vi "MAIN.vi"() -> ()   [LabVIEW 2017]
doc: "该模板用于创建生产者／消费者模式的应用程序，以事件驱动的方式，生成队列中的项。如需通过响应事件实现代码的异步执行，同时不影响用户界面的响应速度，可考虑用该模式替代“用户界面事件处理器”模式。"
uses:
  SubVIs/ctl/Status.ctl
  SubVIs/DataBaseModule/Sqlite/CBB/UpdateAllData.vi
  SubVIs/DataBaseModule/Sqlite/SQLite.lvlib
panel:
  out "stripped path":path
  out "设备Status":T1[](array[typedef])
  in  "设备明细簇":T2[](array[typedef])
  out "元素":string
  in  "选项卡控件":enum32{"主界面", "设置"}(tab)
  out "系统信息":string
  out "Status":T1
  in  "设备名称":T3
  in  "stop":bool caption="停止"
  in  "应用名称":string="InoTouchPad"
  in  "设备明细表格":string[][](table)
  in  "单台设备明细":T2
  out "数据输出":string
  in  "Enqueue Element":bool caption="元素入队列"
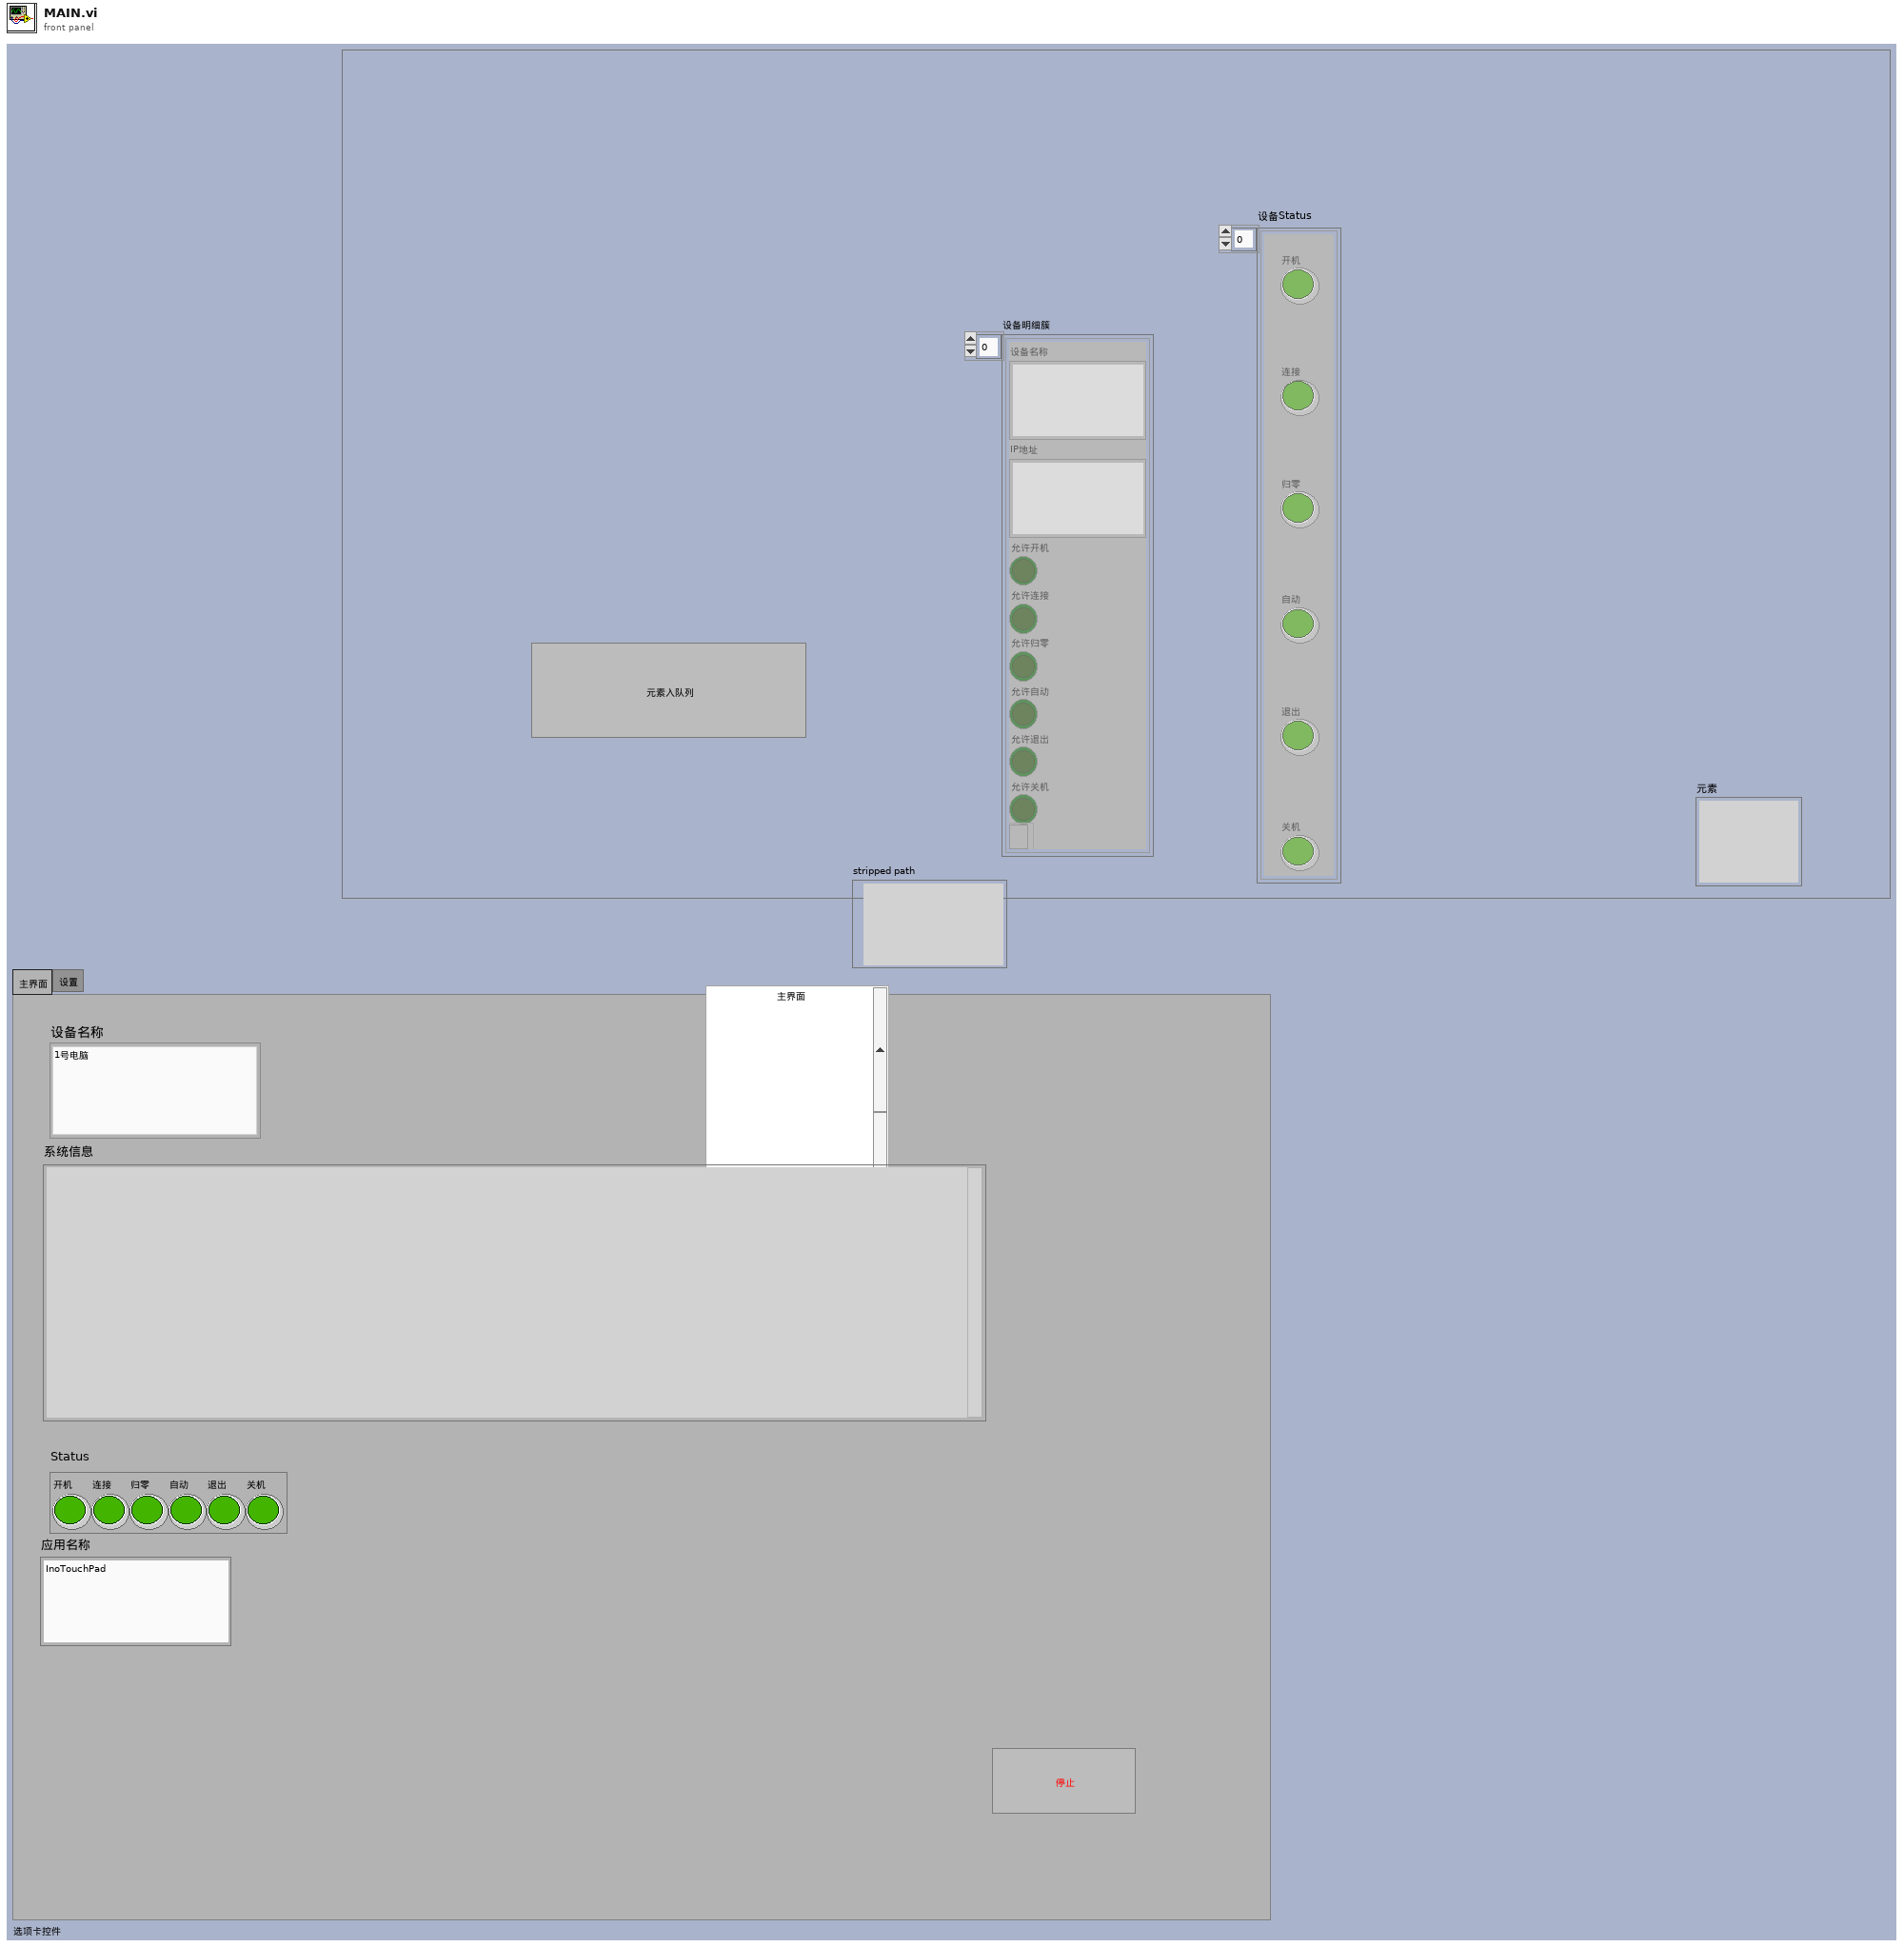
[diagram p1: front panel]
types:
  T1 = typedef "Status.ctl" = cluster{"开机":bool, "连接":bool, "归零":bool, "自动":bool, "退出":bool, "关机":bool}
  T2 = typedef "单台设备明细.ctl" = cluster{"设备名称":string, "IP地址":string, "允许开机":bool, "允许连接":bool, "允许归零":bool, "允许自动":bool, "允许退出":bool, "允许关机":bool, "connection ID":refnum<k5>}
  T3 = typedef "设备名称.ctl" = enum16{"1号电脑", "2号电脑"}
  T4 = enum32{"invalid app kind", "Development System", "Run Time System", "Student Edition", "Embedded LabVIEW", "Evaluation", "Custom"}
  T5 = typedef "界面控件引用.ctl" = cluster{"设备名称":refnum<vi>, "Status":refnum<vi>, "设备明细表格":refnum<vi>, "系统信息":refnum<vi>, "设备明细簇":refnum<vi>, "设备Status":refnum<vi>, "单台设备明细":refnum<vi>}
  T6 = cluster{"设备明细":cluster{"table":string, "column":string[]}, "ER":cluster{"table":string, "column":string[]}}
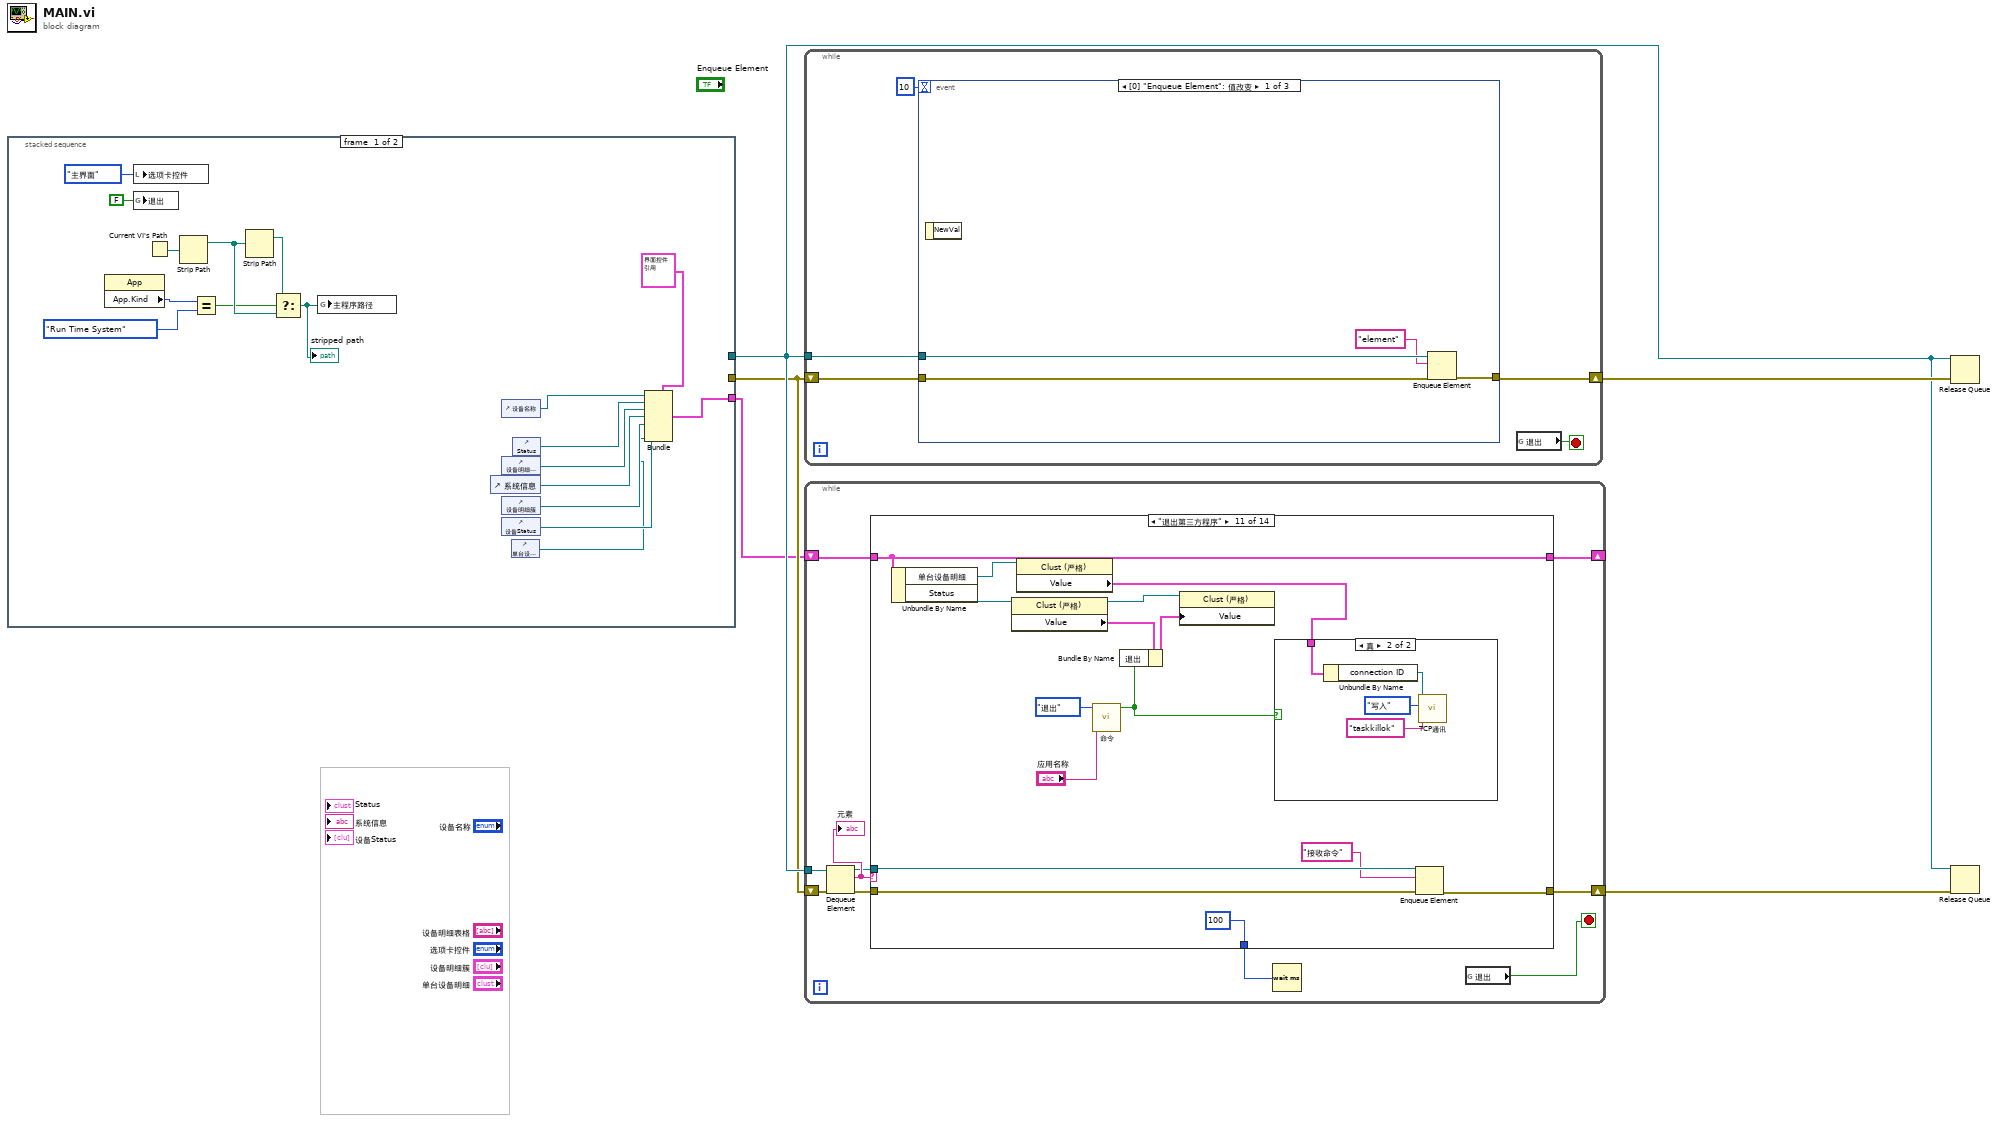
[diagram p0: block diagram]
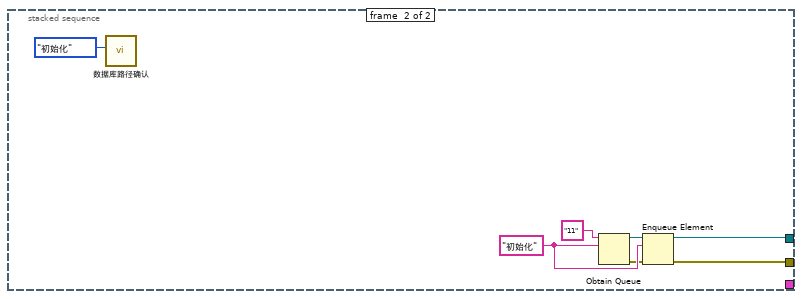
[diagram p2: hidden frame]
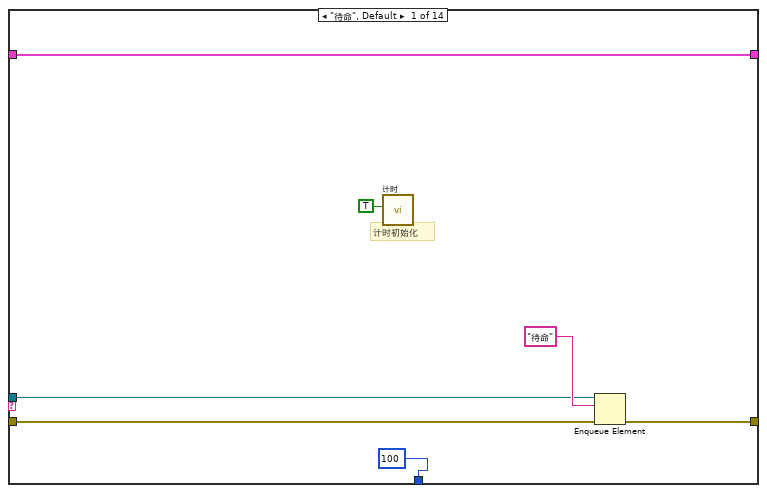
[diagram p3: hidden frame]
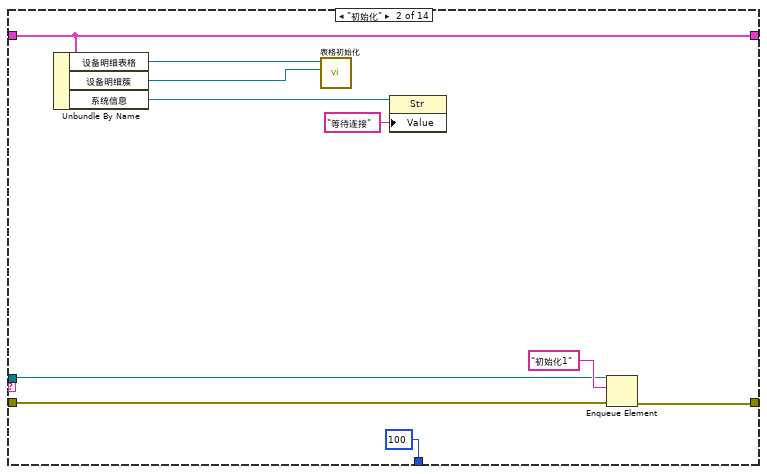
[diagram p4: hidden frame]
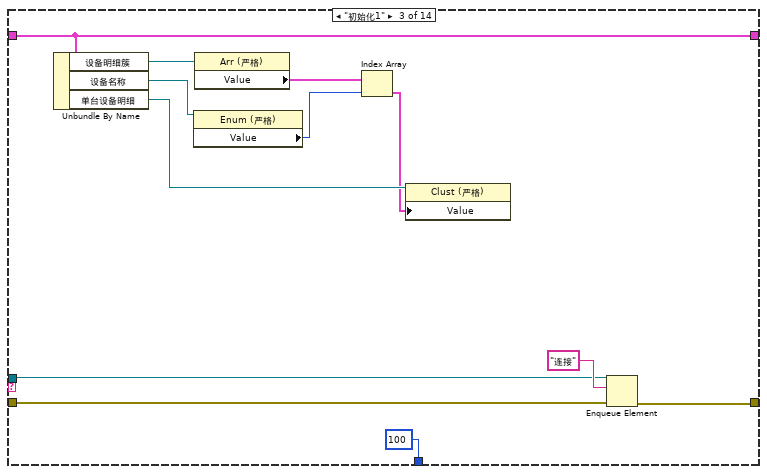
[diagram p5: hidden frame]
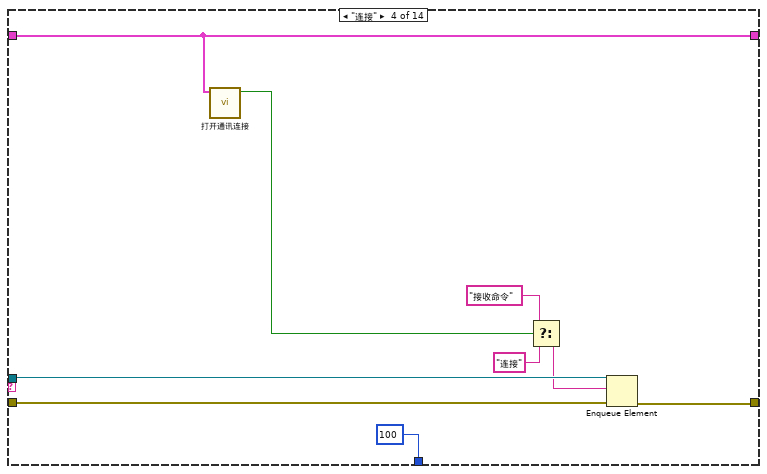
[diagram p6: hidden frame]
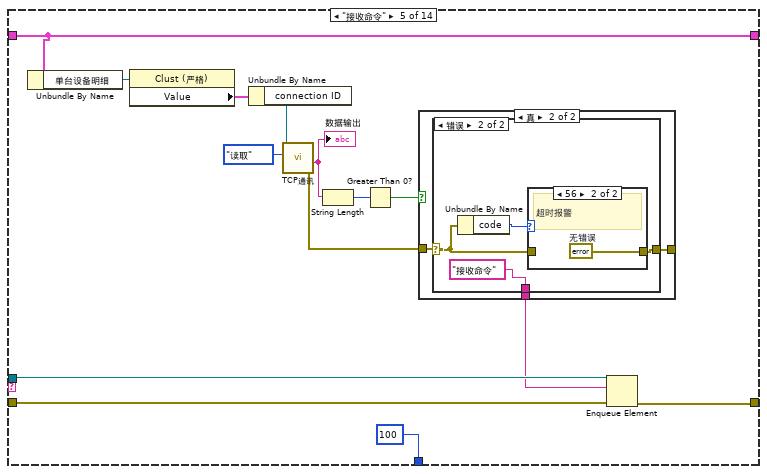
[diagram p7: hidden frame]
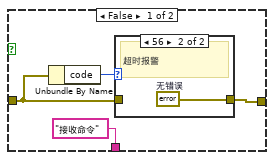
[diagram p8: hidden frame]
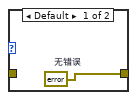
[diagram p9: hidden frame]
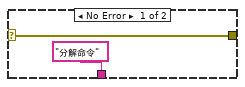
[diagram p10: hidden frame]
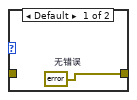
[diagram p11: hidden frame]
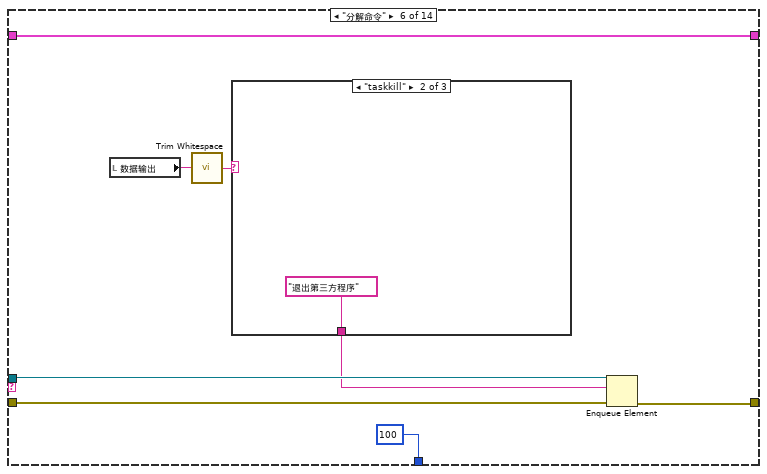
[diagram p12: hidden frame]
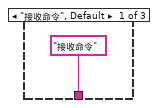
[diagram p13: hidden frame]
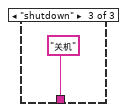
[diagram p14: hidden frame]
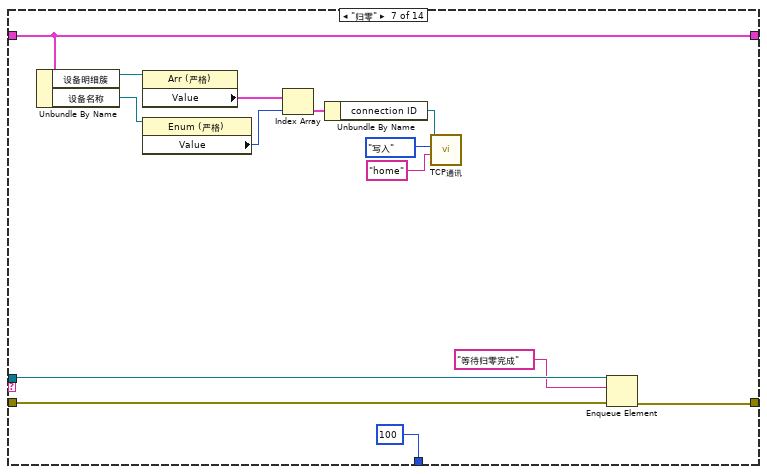
[diagram p15: hidden frame]
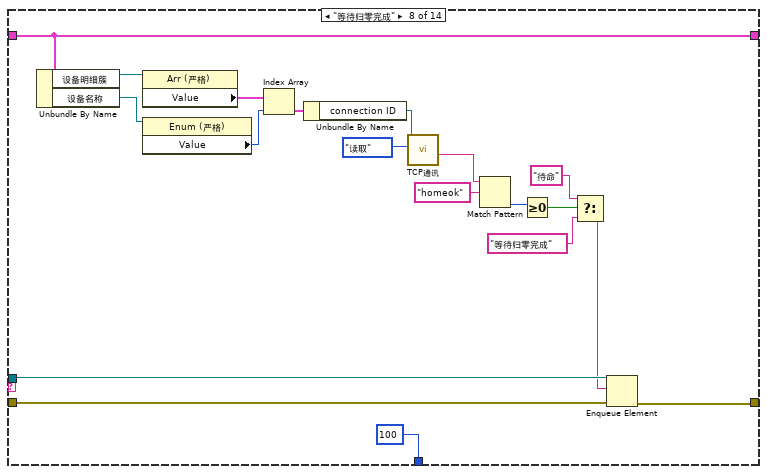
[diagram p16: hidden frame]
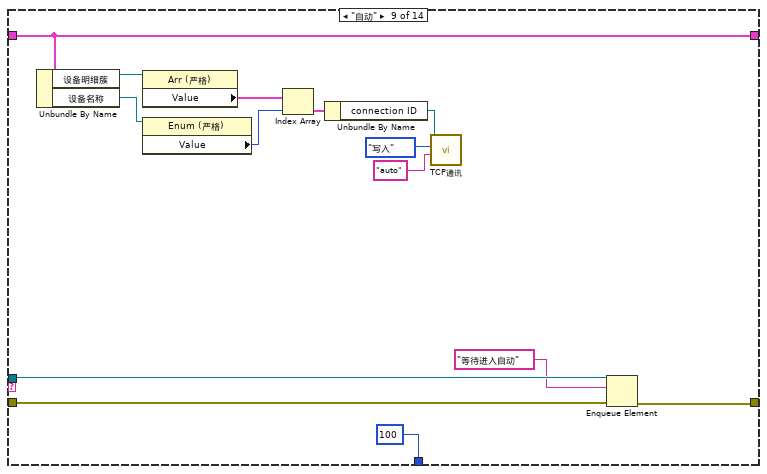
[diagram p17: hidden frame]
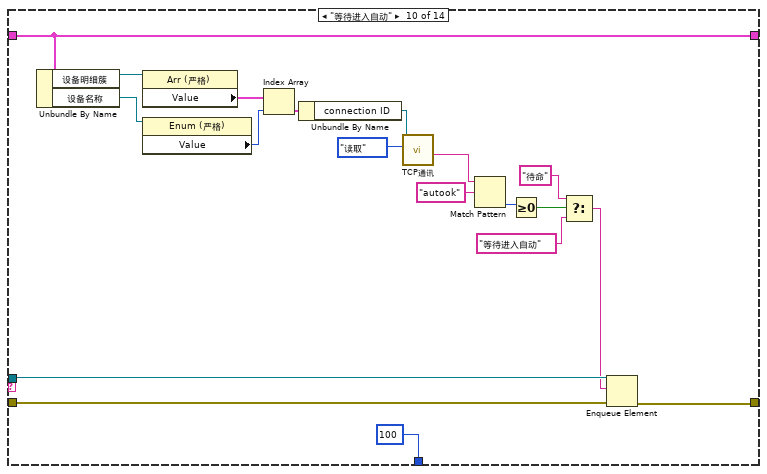
[diagram p18: hidden frame]
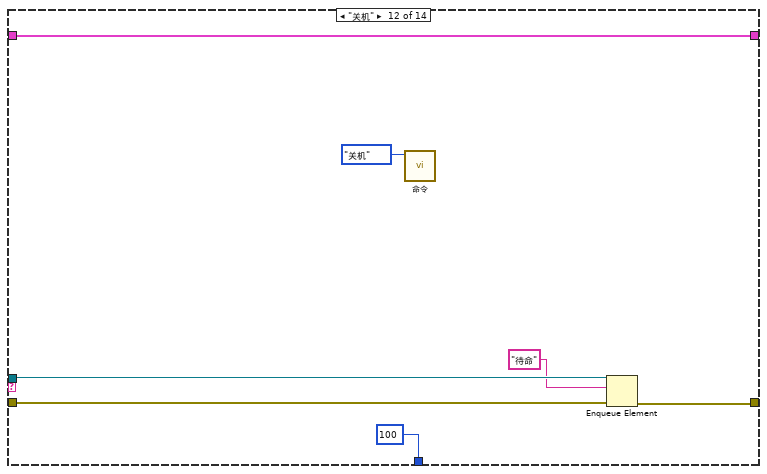
[diagram p20: hidden frame]
diagram:
  n1 = stacked-sequence {
    tunnel: [_ w25] -> w3
    tunnel: [_ w28] -> w4
    tunnel: [w19 _] -> w1
    frame #0 {
      n2 = property class="App"() -> ("App.Kind"=w11:T4)  [unwired: 2 in, 2 out]
      n3 = local write "选项卡控件"(enum32{"主界面", "设置"}."主界面" ("选项卡控件 2")) -> ()
      n4 = global write "全局 1.vi" "退出"(FALSE ("退出")) -> ()
      n5 = Current VI's Path() -> (path=w10:path)
      n6 = Strip Path(path=w10) -> (stripped path=w12:path)  [unwired: 1 out]
      n7 = Equal?(x=w11, y=T4."Run Time System") -> (x = y?=w9:bool)
      n8 = Strip Path(path=w12) -> (stripped path=w8:path)  [unwired: 1 out]
      n9 = Select(t=w8, s=w9, f=w12) -> (s? t:f=w7:path)
      "stripped path" <- w7
      n10 = global write "全局 1.vi" "主程序路径"(w7) -> ()
      n11 = control-ref of="系统信息"() -> (w17:refnum<vi>)
      n12 = control-ref of="设备名称"() -> (w21:refnum<vi>)
      n13 = control-ref of="设备明细表格"() -> (w18:refnum<vi>)
      n14 = control-ref of="设备明细簇"() -> (w16:refnum<vi>)
      n15 = control-ref of="设备Status"() -> (w15:refnum<vi>)
      n16 = control-ref of="单台设备明细"() -> (w14:refnum<vi>)
      n17 = control-ref of="Status"() -> (w20:refnum<vi>)
      n18 = Bundle(cluster=T5 {"设备名称"=refnum, "Status"=refnum, "设备明细表格"=refnum, "系统信息"=refnum, "设备明细簇"=refnum, "设备Status"=refnum, "单台设备明细"=refnum} ("输出簇"), "设备名称"=w21, "Status"=w20, "设备明细表格"=w18, "系统信息"=w17, "设备明细簇"=w16, "设备Status"=w15, "单台设备明细"=w14) -> (w19:T5)
    }
    frame #1 {
      w27 = "初始化"
      n19 = call "数据库路径确认.vi"("选项"=enum16{"初始化", "读取"}."初始化") -> ()  [unwired: 10 in, 1 out]
      n20 = Obtain Queue(name (unnamed)="11" ("名称（未命名）"), element data type=w27) -> (queue out=w30:refnum<queue>, error out=w26:errorcluster)  [unwired: 3 in, 1 out]
      n21 = Enqueue Element(queue=w30, element=w27, error in (no error)=w26) -> (queue out=w28:refnum<queue>, error out=w25:errorcluster)  [unwired: 1 in, 1 out]
    }
  }
  n22 = while {
    shift-right: [w33] -> w5
    shift-left: w3 -> [w34]
    tunnel: w4 -> [w35]
    stop <- w31 stop-if-true
    n23 = event shown="[0] \"Enqueue Element\": 值改变" {
      selector: _ -> [_ _ _]
      dyn-events: _ -> [_ _ _]
      timeout: 10 -> [_ _ _]
      tunnel: w35 -> [w39 _ w44]
      tunnel: w34 -> [w38 _ w42]
      tunnel: [w37 _ w41] -> w33
      event "Enqueue Element": Value Change {
        n24 = event-data() -> ()  [unwired: 1 in, 1 out]
        n25 = Enqueue Element(queue=w39, element="element", error in (no error)=w38) -> (error out=w37:errorcluster)  [unwired: 1 in, 2 out]
      }
      event Timeout {
        n26 = event-data() -> ()  [unwired: 1 in, 3 out]
      }
      event "stop": Value Change {
        n27 = event-data() -> ()  [unwired: 1 in, 1 out]
        n28 = Flush Queue(queue=w44) -> (queue out=w40:refnum<queue>)  [unwired: 1 in, 2 out]
        n29 = Enqueue Element At Opposite End(queue=w40, element="停止" ("元素"), error in (no error)=w42) -> (error out=w41:errorcluster)  [unwired: 1 in, 2 out]
      }
    }
    n30 = global read "全局 1.vi" "退出"() -> (w31:bool)
  }
  n31 = while {
    shift-right: [w50] -> _
    shift-left: w1 -> [w49]
    tunnel: w4 -> [w54]
    shift-right: [w47] -> w2
    shift-left: w3 -> [w48]
    stop <- w46 stop-if-true
    n32 = Dequeue Element(queue=w54, error in (no error)=w48) -> (queue out=w51:refnum<queue>, element=w53:string, error out=w52:errorcluster)  [unwired: 1 in, 1 out]
    "元素" <- w53
    n33 = case shown="\"退出第三方程序\"" w53 {
      tunnel: w52 -> [w58 w71 w83 w92 w106 w131 w148 w167 w181 w200 w215 w226 w241 w255]
      tunnel: [w56 w69 w81 w91 w105 w130 w147 w166 w180 w199 w214 w225 w240 w263] -> w47
      tunnel: w51 -> [w57 w68 w80 w90 w104 w129 w146 w165 w179 w198 w213 w224 w239 w264]
      tunnel: [w61 w66 w78 w84 w101 w127 w143 w163 w176 w196 w209 w221 w234 w260] -> w50
      tunnel: w49 -> [w61 w66 w78 w84 w101 w127 w143 w163 w176 w196 w209 w221 w234 w260]
      tunnel: [u32 100 ("等待时间（毫秒）") u32 100 ("等待时间（毫秒）") u32 100 ("等待时间（毫秒）") u32 100 ("等待时间（毫秒）") u32 100 ("等待时间（毫秒）") u32 100 ("等待时间（毫秒）") u32 100 ("等待时间（毫秒）") u32 100 ("等待时间（毫秒）") u32 100 ("等待时间（毫秒）") u32 100 ("等待时间（毫秒）") u32 100 ("等待时间（毫秒）") u32 100 ("等待时间（毫秒）") u32 100 ("等待时间（毫秒）") u32 100 ("等待时间（毫秒）")] -> w45
      frame "待命", Default {
        # "计时初始化"
        n34 = call "计时.vi"("初始化"=TRUE) -> ()  [unwired: 9 in, 2 out]
        n35 = Enqueue Element(queue=w57, element="待命", error in (no error)=w58) -> (error out=w56:errorcluster)  [unwired: 1 in, 2 out]
      }
      frame "初始化" {
        n36 = Unbundle By Name(w66) -> ("设备明细表格"=w65:refnum<vi>, "设备明细簇"=w64:refnum<vi>, "系统信息"=w63:refnum<vi>)
        n37 = call "表格初始化.vi"("设备明细簇"=w64, "Table输入"=w65) -> ()  [unwired: 10 in]
        n38 = property class="Str"(reference=w63, "Value"="等待连接" ("值")) -> ()  [unwired: 1 in, 2 out]
        n39 = Enqueue Element(queue=w68, element="初始化1", error in (no error)=w71) -> (error out=w69:errorcluster)  [unwired: 1 in, 2 out]
      }
      frame "初始化1" {
        n40 = Unbundle By Name(w78) -> ("设备明细簇"=w76:refnum<vi>, "设备名称"=w75:refnum<vi>, "单台设备明细"=w77:refnum<vi>)
        n41 = property class="Enum (严格)"(reference=w75) -> ("Value"=w73:T3)  [unwired: 1 in, 2 out]
        n42 = property class="Arr (严格)"(reference=w76) -> ("Value"=w74:T2[])  [unwired: 1 in, 2 out]
        n43 = Index Array(array=w74, index=w73) -> (element=w72:T2)
        n44 = property class="Clust (严格)"(reference=w77, "Value"=w72) -> ()  [unwired: 1 in, 2 out]
        n45 = Enqueue Element(queue=w80, element="连接", error in (no error)=w83) -> (error out=w81:errorcluster)  [unwired: 1 in, 2 out]
      }
      frame "连接" {
        n46 = call "打开通讯连接.vi"("界面控件引用"=w84) -> ("连接成功"=w86:bool)  [unwired: 10 in]
        n47 = Select(t="接收命令", s=w86, f="连接" ("t")) -> (s? t:f=w87:string)
        n48 = Enqueue Element(queue=w90, element=w87, error in (no error)=w92) -> (error out=w91:errorcluster)  [unwired: 1 in, 2 out]
      }
      frame "接收命令" {
        n49 = Unbundle By Name(w101) -> ("单台设备明细"=w100:refnum<vi>)
        n50 = property class="Clust (严格)"(reference=w100) -> ("Value"=w99:T2)  [unwired: 1 in, 2 out]
        n51 = Unbundle By Name(w99) -> ("connection ID"=w102:refnum<k5>)
        n52 = call "TCP通讯.vi"("选项"=enum16{"NA", "侦听", "读取", "写入", "关闭", "打开TCP连接"}."读取", "connection ID in"=w102) -> ("error out"=w94:errorcluster, "数据输出"=w96:string)  [unwired: 5 in, 3 out]
        "数据输出" <- w96
        n53 = String Length(string=w96) -> (length=w95:i32)
        n54 = Greater Than 0?(x=w95) -> (x > 0?=w97:bool)
        n55 = case shown="真" w97 {
          tunnel: w94 -> [w109 w115]
          tunnel: [w108 w114] -> _
          tunnel: ["接收命令" ("t") w113] -> w93
          frame False {
            n56 = Unbundle By Name(w109) -> ("code"=w110:i32)
            n57 = case shown="56" w110 {
              tunnel: w109 -> [_ _]
              tunnel: [w111 w112] -> w108
              frame Default {
                w111 = errorcluster {"status"=FALSE, "code"=0, "source"=""}  # 无错误
              }
              frame 56 {
                w112 = errorcluster {"status"=FALSE, "code"=0, "source"=""}  # 无错误
                # "超时报警"
              }
            }
          }
          frame True {
            n58 = case shown="错误" w115 {
              selector: w115 -> [w117 w120]
              tunnel: [w117 w119] -> w114
              tunnel: ["分解命令" ("t") "接收命令" ("t")] -> w113
              frame No Error {
              }
              frame Error {
                n59 = Unbundle By Name(w120) -> ("code"=w121:i32)
                n60 = case shown="56" w121 {
                  tunnel: w120 -> [_ _]
                  tunnel: [w122 w123] -> w119
                  frame Default {
                    w122 = errorcluster {"status"=FALSE, "code"=0, "source"=""}  # 无错误
                  }
                  frame 56 {
                    w123 = errorcluster {"status"=FALSE, "code"=0, "source"=""}  # 无错误
                    # "超时报警"
                  }
                }
              }
            }
          }
        }
        n61 = Enqueue Element(queue=w104, element=w93, error in (no error)=w106) -> (error out=w105:errorcluster)  [unwired: 1 in, 2 out]
      }
      frame "分解命令" {
        n62 = local read "数据输出"() -> (w125:string)
        n63 = call <vilib>:"Trim Whitespace.vi"("string"=w125) -> ("trimmed string"=w124:string)  [unwired: 1 in]
        n64 = case shown="\"taskkill\"" w124 {
          tunnel: ["接收命令" ("t") "退出第三方程序" ("t") "关机" ("t")] -> w126
          frame "接收命令", Default {
          }
          frame "taskkill" {
          }
          frame "shutdown" {
          }
        }
        n65 = Enqueue Element(queue=w129, element=w126, error in (no error)=w131) -> (error out=w130:errorcluster)  [unwired: 1 in, 2 out]
      }
      frame "归零" {
        n66 = Unbundle By Name(w143) -> ("设备明细簇"=w142:refnum<vi>, "设备名称"=w140:refnum<vi>)
        n67 = property class="Arr (严格)"(reference=w142) -> ("Value"=w138:T2[])  [unwired: 1 in, 2 out]
        n68 = property class="Enum (严格)"(reference=w140) -> ("Value"=w137:T3)  [unwired: 1 in, 2 out]
        n69 = Index Array(array=w138, index=w137) -> (element=w139:T2)
        n70 = Unbundle By Name(w139) -> ("connection ID"=w136:refnum<k5>)
        n71 = call "TCP通讯.vi"("数据输入"="home", "选项"=enum16{"NA", "侦听", "读取", "写入", "关闭"}."写入", "connection ID in"=w136) -> ()  [unwired: 4 in, 5 out]
        n72 = Enqueue Element(queue=w146, element="等待归零完成" ("t"), error in (no error)=w148) -> (error out=w147:errorcluster)  [unwired: 1 in, 2 out]
      }
      frame "等待归零完成" {
        n73 = Unbundle By Name(w163) -> ("设备明细簇"=w162:refnum<vi>, "设备名称"=w160:refnum<vi>)
        n74 = property class="Arr (严格)"(reference=w162) -> ("Value"=w158:T2[])  [unwired: 1 in, 2 out]
        n75 = property class="Enum (严格)"(reference=w160) -> ("Value"=w157:T3)  [unwired: 1 in, 2 out]
        n76 = Index Array(array=w158, index=w157) -> (element=w159:T2)
        n77 = Unbundle By Name(w159) -> ("connection ID"=w156:refnum<k5>)
        n78 = call "TCP通讯.vi"("选项"=enum16{"NA", "侦听", "读取", "写入", "关闭"}."读取", "connection ID in"=w156) -> ("数据输出"=w155:string)  [unwired: 5 in, 4 out]
        n79 = Match Pattern(string=w155, regular expression="homeok" ("正则表达式")) -> (offset past match=w153:i32)  [unwired: 1 in, 3 out]
        n80 = Greater Or Equal To 0?(x=w153) -> (x >= 0?=w152:bool)
        n81 = Select(t="待命", s=w152, f="等待归零完成" ("t")) -> (s? t:f=w150:string)
        n82 = Enqueue Element(queue=w165, element=w150, error in (no error)=w167) -> (error out=w166:errorcluster)  [unwired: 1 in, 2 out]
      }
      frame "自动" {
        n83 = Unbundle By Name(w176) -> ("设备明细簇"=w175:refnum<vi>, "设备名称"=w173:refnum<vi>)
        n84 = property class="Arr (严格)"(reference=w175) -> ("Value"=w171:T2[])  [unwired: 1 in, 2 out]
        n85 = property class="Enum (严格)"(reference=w173) -> ("Value"=w170:T3)  [unwired: 1 in, 2 out]
        n86 = Index Array(array=w171, index=w170) -> (element=w172:T2)
        n87 = Unbundle By Name(w172) -> ("connection ID"=w169:refnum<k5>)
        n88 = call "TCP通讯.vi"("数据输入"="auto", "选项"=enum16{"NA", "侦听", "读取", "写入", "关闭"}."写入", "connection ID in"=w169) -> ()  [unwired: 4 in, 5 out]
        n89 = Enqueue Element(queue=w179, element="等待进入自动" ("t"), error in (no error)=w181) -> (error out=w180:errorcluster)  [unwired: 1 in, 2 out]
      }
      frame "等待进入自动" {
        n90 = Unbundle By Name(w196) -> ("设备明细簇"=w195:refnum<vi>, "设备名称"=w193:refnum<vi>)
        n91 = property class="Arr (严格)"(reference=w195) -> ("Value"=w191:T2[])  [unwired: 1 in, 2 out]
        n92 = property class="Enum (严格)"(reference=w193) -> ("Value"=w190:T3)  [unwired: 1 in, 2 out]
        n93 = Index Array(array=w191, index=w190) -> (element=w192:T2)
        n94 = Unbundle By Name(w192) -> ("connection ID"=w189:refnum<k5>)
        n95 = call "TCP通讯.vi"("选项"=enum16{"NA", "侦听", "读取", "写入", "关闭"}."读取", "connection ID in"=w189) -> ("数据输出"=w188:string)  [unwired: 5 in, 4 out]
        n96 = Match Pattern(string=w188, regular expression="autook" ("正则表达式")) -> (offset past match=w186:i32)  [unwired: 1 in, 3 out]
        n97 = Greater Or Equal To 0?(x=w186) -> (x >= 0?=w185:bool)
        n98 = Select(t="待命", s=w185, f="等待进入自动" ("t")) -> (s? t:f=w183:string)
        n99 = Enqueue Element(queue=w198, element=w183, error in (no error)=w200) -> (error out=w199:errorcluster)  [unwired: 1 in, 2 out]
      }
      frame "退出第三方程序" {
        n100 = Unbundle By Name(w209) -> ("单台设备明细"=w204:refnum<vi>, "Status"=w208:refnum<vi>)
        n101 = property class="Clust (严格)"(reference=w208) -> (reference out=w207:refnum<vi>, "Value"=w206:T1)  [unwired: 1 in, 1 out]
        n102 = property class="Clust (严格)"(reference=w204) -> ("Value"=w203:T2)  [unwired: 1 in, 2 out]
        n103 = call "命令.vi"("应用名称"="应用名称", "选项"=enum16{"归零", "自动", "退出", "关机"}."退出") -> ("完成"=w202:bool)  [unwired: 9 in]
        n104 = Bundle By Name(cluster=w206, "退出"=w202) -> (w205:T1)
        n105 = property class="Clust (严格)"(reference=w207, "Value"=w205) -> ()  [unwired: 1 in, 2 out]
        n106 = case shown="真" w202 {
          tunnel: w203 -> [_ w218]
          frame False {
          }
          frame True {
            n107 = Unbundle By Name(w218) -> ("connection ID"=w219:refnum<k5>)
            n108 = call "TCP通讯.vi"("数据输入"="taskkillok", "选项"=enum16{"NA", "侦听", "读取", "写入", "关闭", "打开TCP连接"}."写入", "connection ID in"=w219) -> ()  [unwired: 4 in, 5 out]
          }
        }
        n109 = Enqueue Element(queue=w213, element="接收命令" ("t"), error in (no error)=w215) -> (error out=w214:errorcluster)  [unwired: 1 in, 2 out]
      }
      frame "关机" {
        n110 = call "命令.vi"("选项"=enum16{"归零", "自动", "退出", "关机"}."关机") -> ()  [unwired: 10 in, 1 out]
        n111 = Enqueue Element(queue=w224, element="待命" ("t"), error in (no error)=w226) -> (error out=w225:errorcluster)  [unwired: 1 in, 2 out]
      }
      frame "保存" {
        n112 = Unbundle By Name(w234) -> ("设备明细表格"=w236:refnum<vi>)
        n113 = property class="Tbl (严格)"(reference=w236) -> (reference out=w233:refnum<vi>, "Value"=w232:string[][])  [unwired: 1 in, 1 out]
        n114 = in-place {
          in-place-border: w232 -> [w244]
          in-place-border: [w243] -> w228
          in-place-border: [w242] -> w227
          n115 = for {
            tunnel: w244 -> [w253] mode=indexing
            tunnel: [w253] -> w243 mode=indexing if=w249
            # "删除空白项"
            n116 = Index Array(array=w253, index=2 ("禁用的索引 (列)")) -> (element=w251:string)
            n117 = Empty String/Path?(string/path=w251) -> (empty?=w250:bool)
            n118 = Not(x=w250) -> (.not. x?=w249:bool)
          }
          n119 = for {
            tunnel: w243 -> [w246] mode=indexing
            tunnel: [w245] -> w242 mode=indexing
            n120 = for {
              tunnel: w246 -> [w248] mode=indexing
              tunnel: [w247] -> w245 mode=indexing
              n121 = Text to UTF-8(11:w248) -> (3:w247:string)  [unwired: 2 in, 1 out]
            }
          }
        }
        n122 = call "tables&columns.vi"("选项"=enum16{"初始化", "获取寄存器"}."获取寄存器") -> ("Tables&columns"=w230:T6)  [unwired: 9 in, 1 out]
        n123 = Unbundle By Name(w230) -> ("设备明细.table"=w229:string)
        n124 = call "数据库路径确认.vi"() -> ("数据库路径"=w235:path)  [unwired: 11 in]
        n125 = property class="Tbl (严格)"(reference=w233, "Value"=w228) -> ()  [unwired: 1 in, 2 out]
        n126 = Enqueue Element(queue=w239, element="待命" ("t"), error in (no error)=w241) -> (error out=w240:errorcluster)  [unwired: 1 in, 2 out]
        n127 = call-poly "SQLite多态.vi"("AllData"=w227, "Table Name"=w229, "DbPath"=w235) -> ()  [unwired: 5 in, 4 out]
      }
      frame "停止" {
        n128 = Unbundle By Name(w260) -> ("单台设备明细"=w259:refnum<vi>)
        n129 = property class="Clust (严格)"(reference=w259) -> ("Value"=w258:T2)  [unwired: 1 in, 2 out]
        n130 = Unbundle By Name(w258) -> ("connection ID"=w257:refnum<k5>)
        n131 = call "TCP通讯.vi"("error in"=w255, "选项"=enum16{"NA", "侦听", "读取", "写入", "关闭", "打开TCP连接"}."关闭", "connection ID in"=w257) -> ("error out"=w254:errorcluster)  [unwired: 4 in, 4 out]
        n132 = Flush Queue(queue=w264, error in (no error)=w254) -> (error out=w263:errorcluster)  [unwired: 2 out]
        n133 = global write "全局 1.vi" "退出"(TRUE) -> ()
      }
    }
    n134 = Wait (ms)(milliseconds to wait=w45) -> ()  [unwired: 1 out]
    n135 = global read "全局 1.vi" "退出"() -> (w46:bool)
  }
  n136 = Release Queue(queue=w4, error in (no error)=w5) -> ()  [unwired: 1 in, 3 out]
  n137 = Release Queue(queue=w4, error in (no error)=w2) -> ()  [unwired: 1 in, 3 out]
